vi "Constructor_RQMHLogger.vi"(7 "RQMHLogger in":refnum<class "Logger.lvclass">, 8 "error in (no error)":errorcluster, 10 "Handles":refnum<class "HandleHolder.lvclass">[](array[class]), 11 "Name (Logger)":string="Logger") -> (0 "error out":errorcluster, 3 "RQMHLogger out":refnum<class "Logger.lvclass">)   [LabVIEW 2024, in "Logger.lvclass"]
uses:
  Logger.lvclass
  HandleHolder/HandleHolder.lvclass
  Logger.lvclass/Logger.ctl
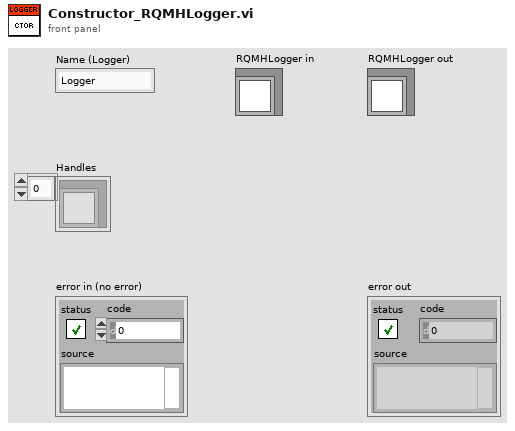
[diagram p1: front panel]
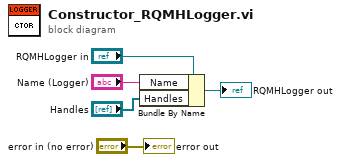
[diagram p0: block diagram]
diagram:
  n1 = Bundle By Name(cluster="RQMHLogger in", "Name"="Name (Logger)", "Handles"="Handles") -> (→"RQMHLogger out":refnum<class "Logger.lvclass">)
  "error out" <- "error in (no error)"
